vi "exec.vi"(8 "error in (no error)":errorcluster, 10 "context":refnum<class "Context.lvclass">, 11 "Start in":refnum<class "StartTestScenarioCommand.lvclass">) -> (0 "error out":errorcluster, 2 "context 2":refnum<class "Context.lvclass">, 3 "Start out":refnum<class "StartTestScenarioCommand.lvclass">)   [LabVIEW 2015, in "StartTestScenarioCommand.lvclass"]
uses:
  StartTestScenarioCommand.lvclass
  Context/Context.lvclass
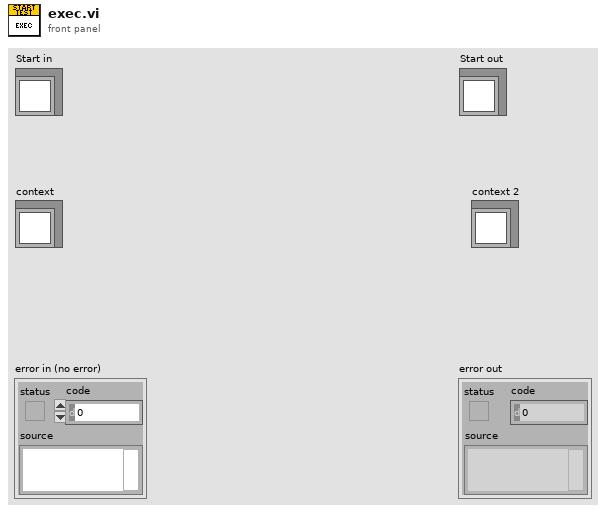
[diagram p1: front panel]
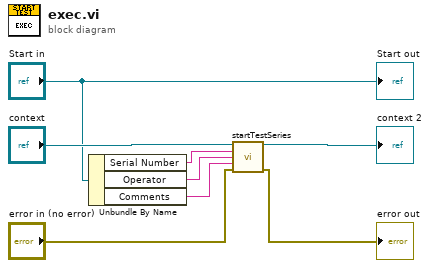
[diagram p0: block diagram]
diagram:
  n1 = Unbundle By Name("Start in") -> ("Serial Number"=w3:string, "Operator"=w2:string, "Comments"=w1:string)
  n2 = call "startTestSeries.vi"("Context in"="context", "Serial Number"=w3, "Operator"=w2, "Comments"=w1, "error in (no error)"="error in (no error)") -> ("Context out"=→"context 2":refnum<class "Context.lvclass">, "error out"=→"error out":errorcluster)  [unwired: 9 in]
  "Start out" <- "Start in"
